vi "Make Command Tag from Name.vi"(10 "Time":dbl, 11 "Cmd Name":string="%.3f secs") -> (3 "Cmd Tag":string)   [LabVIEW 2019]
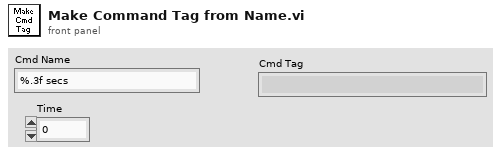
[diagram p1: front panel]
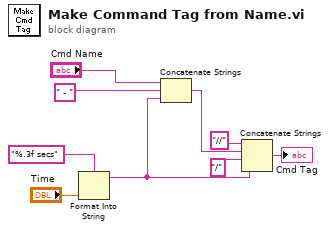
[diagram p0: block diagram]
diagram:
  n1 = Format Into String(format string="%.3f secs", "Time") -> (resulting string=w4:string)  [unwired: 2 in, 1 out]
  n2 = Concatenate Strings("Cmd Name", " - ", w4) -> (w1:string)
  n3 = Concatenate Strings("//", w1, "/", w4) -> (→"Cmd Tag":string)
